vi "Shared Variables CD 2.0 GUID Lookup.vi"() -> ()   [LabVIEW 2017]
doc: "Use this Global VI to access the GUIDs assigned to the page resources of the Custom Device."
panel:
  in  "Error Page":string="5436e1eb-8f7b-49f2-9830-32976c323e56"
  in  "Status Page":string="bf290bea-42ed-4a60-879f-a311dbe4de0f"
  in  "Boolean Page":string="5e384cd8-807c-47a7-a973-215c0a8952b3"
  in  "Numeric Page":string="5480142c-f7e0-4c41-8ce2-b6ae3e17b247"
  in  "Target Page":string="9bbfc2a2-d0f2-430a-9bec-35d10b28e45e"
  in  "Read Page":string="4fe9b085-dccc-493b-bd60-f87426b0df9b"
  in  "Write Page":string="03ebf737-a43a-4cae-9229-a600a1cb01e1"
  in  "Custom Device Page":string="e36672b6-b061-4dec-a686-6b6cf69ca646"
  # "GUID for Pages"
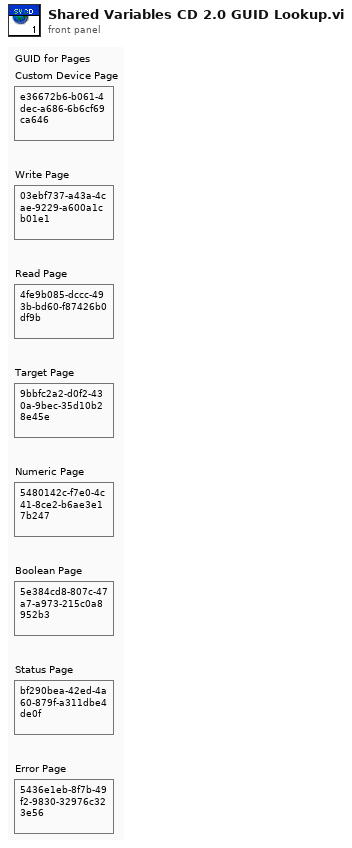
[diagram p1: front panel]
diagram:
